vi "DCMotorAccel.vi"() -> ()   [LabVIEW 2018]
uses:
  <vilib>/Platform/TimedLoop/XDataNode/timing_clust.ctl
  <vilib>/Platform/TimedLoop/XDataNode/nitl_modes.ctl
  <vilib>/Platform/TimedLoop/XDataNode/wakeup.ctl
  <vilib>/MakerHub/LINX/Public/Utilities/Open Serial.vi
  <vilib>/MakerHub/LINX/Public/Sensors/Motion/Servo/Servo Set Pulse Width One Channel.vi
  <vilib>/MakerHub/LINX/Public/Sensors/Motion/Servo/Servo Close One Channel.vi
  <vilib>/platform/TimedLoop/XDataNode/XDataNode.xnode
  <vilib>/MakerHub/LINX/Public/Sensors/Motion/Servo/Servo Open One Channel.vi
  <vilib>/MakerHub/LINX/LMH-LINX.lvlib
  <vilib>/MakerHub/LINX/Public/Sensors/Motion/Servo/Servo.lvlib
  <vilib>/Platform/TimedLoop/XDataNode/XDNodeRunTimeDep.lvlib
panel:
  in  "Speed RPM":dbl(knob) scale=-100.0..100.0
  in  "Acceleration RPM/ms":dbl(knob) scale=0.0..10.0
  in  "Servo Channel":u8
  in  "?":bool
  in  "Baud Rate Override":u32
  in  "Serial Port":refnum<visa-resource-name>="N/A"
  # "Arduino Settings"
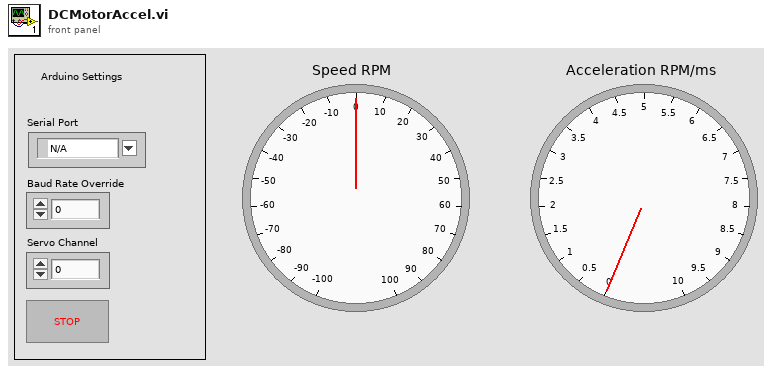
[diagram p1: front panel]
types:
  T1 = typedef "LMH-LINX.lvlib/LINX Ref.ctl" = cluster{"IO":T2, "Interface":T3, "LINX Device Config":T4}
  T2 = typedef "LMH-LINX.lvlib/Platform.ctl" = enum16{"Remote", "Local"}
  T3 = typedef "LMH-LINX.lvlib/Interface.ctl" = enum16{"Serial", "TCP"}
  T4 = typedef "LMH-LINX.lvlib/Device.lvlib/LINX Device Config.ctl" = cluster{"Interface":T3, "COM Port":refnum<visa-resource-name>, "TCP Configuration":T5, "Device Family":u8, "Device ID":u8, "Device Name":string, "TCP Ref":refnum<k5>, "Channels":T6}
  T5 = typedef "LMH-LINX.lvlib/Device.lvlib/TCP Config.ctl" = cluster{"IP Address":string, "Port":u16}
  T6 = typedef "LMH-LINX.lvlib/Channels.ctl" = cluster{"DI":u8[], "DO":u8[], "AI":u8[], "AO":u8[], "PWM":u8[], "QE":u8[], "UART":u8[], "I2C 2":u8[], "SPI":u8[], "CAN":u8[], "Servo":u8[], "AI Ref (V)":dbl, "AI Resolution (Bits)":u8, "AO Ref (V)":dbl, "AO Resolution (Bits)":u8}
  T7 = typedef "XDNodeRunTimeDep.lvlib/timing_clust.ctl" = cluster{"Expected End [f-1]":u64, "Actual End [f-1]":u64, "Finished Late? [f-1]":bool, "Expected End [i-1]":u64, "Actual End [i-1]":u64, "Finished Late? [i-1]":bool, "Expected Start [i]":u64, "Actual Start [i]":u64, "Expected Start [f]":u64, "Actual Start [f]":u64, "Source Name":string, "Structure Name":string, "Period":i64, "Deadline":i64, "Offset":i64, "Start":i64, "Priority":i32, "Timeout":i32, "Mode":T8, "Wakeup Reason":T9, "Error":errorcluster, "Source Type":string, "Secondary Source Type":string, "Global End Time":u64, "Global Start Time":u64, "Frame Duration":u64, "Iteration Duration":u64, "Assigned CPU":i32, "I/O Scan Engine Mode":u32}
  T8 = typedef "XDNodeRunTimeDep.lvlib/nitl_modes.ctl" = enum32{"No Change", "Process missed periods, maintain original phase", "Discard missed periods, maintain original phase", "Process missed periods, ignore original phase", "Discard missed periods, ignore original phase"}
  T9 = typedef "XDNodeRunTimeDep.lvlib/wakeup.ctl" = enum32{"Normal", "Aborted", "Asynchronous wakeup", "Timing source error", "Timed loop error", "Timeout"}
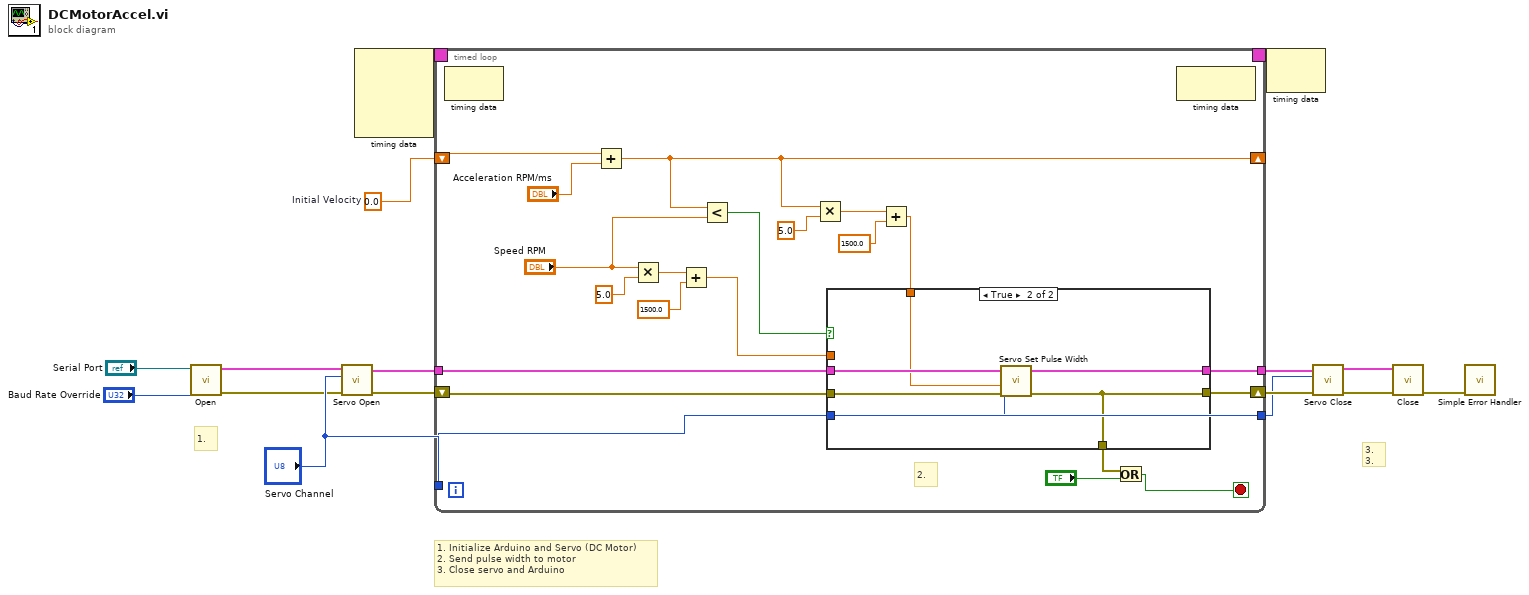
[diagram p0: block diagram]
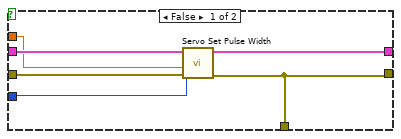
[diagram p2: hidden frame]
diagram:
  w4 = 0.0  # Initial Velocity
  # "1. Initialize Arduino and Servo (DC Motor)\n2. Send pulse width to motor\n3. Close servo and Arduino"
  # "3.\n3."
  # "1."
  n1 = call-poly <vilib>:"Open.vi"("Baud Rate Override"="Baud Rate Override", "Serial Port"="Serial Port") -> ("Error Out"=w5:errorcluster, "LINX Resource"=w6:T1)  [unwired: 7 in, 1 out]
  n2 = call-poly <vilib>:"Servo Open.vi"("Error In"=w5, "Servo Channel"="Servo Channel", "LINX Resource"=w6) -> ("Error Out"=w12:errorcluster, "LINX Resource"=w13:T1)  [unwired: 7 in]
  n3 = node-c288() -> (w2:T7)  [unwired: 4 in]
  n4 = timed-loop {
    tunnel: w13 -> [w27]
    tunnel: [w19] -> w11
    shift-right: [w20] -> w10
    shift-left: w12 -> [w26]
    tunnel: "Servo Channel" -> [w17]
    shift-right: [w22] -> _
    shift-left: w4 -> [w34]
    tunnel: [w17] -> w3
    timing: w2 -> [_]
    timing-out: [_] -> w1
    stop <- w37 stop-if-true
    # "2."
    n5 = node-c288() -> ()  [unwired: 1 in, 1 out]
    n6 = Add(x=w34, y="Acceleration RPM/ms") -> (x+y=w22:dbl)
    n7 = Multiply(x="Speed RPM", y=5.0) -> (x*y=w32:dbl)
    n8 = Add(x=w32, y=1500.0) -> (x+y=w28:dbl)
    n9 = Less?(x=w22, y="Speed RPM") -> (x < y?=w33:bool)
    n10 = Multiply(x=w22, y=5.0) -> (x*y=w25:dbl)
    n11 = Add(x=w25, y=1500.0) -> (x+y=w21:dbl)
    n12 = case shown="True" w33 {
      tunnel: w28 -> [w40 _]
      tunnel: w27 -> [w44 w51]
      tunnel: w26 -> [w43 w50]
      tunnel: w17 -> [w45 w49]
      tunnel: [w41 w46] -> w20
      tunnel: w21 -> [_ w48]
      tunnel: [w42 w47] -> w19
      tunnel: [w41 w46] -> w18
      frame False {
        n13 = call-poly <vilib>:"Servo Set Pulse Width.vi"("Error In"=w43, "Pulse Width (uS)"=w40, "Servo Channel"=w45, "LINX Resource"=w44) -> ("Error Out"=w41:errorcluster, "LINX Resource"=w42:T1)  [unwired: 6 in]
      }
      frame True {
        n14 = call-poly <vilib>:"Servo Set Pulse Width.vi"("Error In"=w50, "Pulse Width (uS)"=w48, "Servo Channel"=w49, "LINX Resource"=w51) -> ("Error Out"=w46:errorcluster, "LINX Resource"=w47:T1)  [unwired: 6 in]
      }
    }
    n15 = Or(x=w18, y="?") -> (x .or. y?=w37:bool)
    n16 = node-c288() -> ()  [unwired: 1 in, 1 out]
  }
  n17 = node-c288(w1) -> ()  [unwired: 1 out]
  n18 = call-poly <vilib>:"Servo Close.vi"("Error In"=w10, "Servo Channel"=w3, "LINX Resource"=w11) -> ("Error Out"=w8:errorcluster, "LINX Resource"=w9:T1)  [unwired: 7 in]
  n19 = call <vilib>:"Close.vi"("Error In"=w8, "LINX Resource"=w9) -> ("Error Out"=w14:errorcluster)  [unwired: 9 in]
  n20 = call <vilib>:"Simple Error Handler.vi"("error in (no error)"=w14) -> ()  [unwired: 4 in, 5 out]
